vi "Graphics-Draw Line On Plot.vi"(8 "error in (no error)":errorcluster, 10 "X value":dbl, 11 "XYGraph in":refnum<vi>) -> (0 "error out":errorcluster)   [LabVIEW 2015]
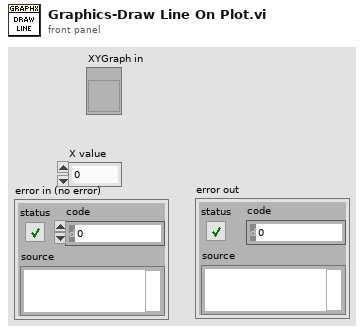
[diagram p1: front panel]
types:
  T1 = cluster{"Width":u16, "Style":enum32{"Solid", "Dash", "Dot", "DashDot", "DashDotDot"}}
  T2 = typedef "LVRectTypeDef.ctl" = cluster{"Left":i16, "Top":i16, "Right":i16, "Bottom":i16}
  T3 = typedef "LVPoint32TypeDef.ctl" = cluster{"Horizontal":i32, "Vertical":i32}
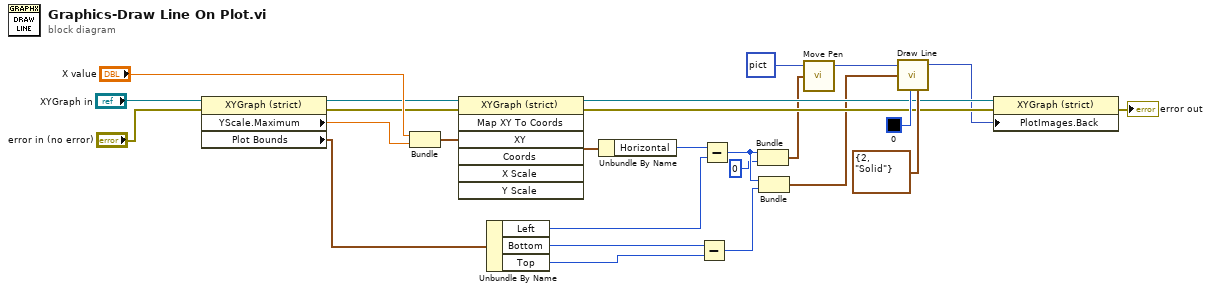
[diagram p0: block diagram]
diagram:
  n1 = property on="Property Node" class="XYGraph (strict)"(reference="XYGraph in", error in="error in (no error)") -> (reference out=w9:refnum<vi>, error out=w13:errorcluster, "YScale.Maximum"=w8:dbl, "Plot Bounds"=w21:T2)
  n2 = Bundle("X value"="X value", "YScale.Maximum"=w8) -> (w17:cluster{"X value":dbl, "YScale.Maximum":dbl})  [unwired: 1 in]
  n3 = invoke on="Invoke Node" class="XYGraph (strict)" method="Map XY To Coords"(reference=w9, error in=w13, "XY"=w17) -> (reference out=w14:refnum<vi>, error out=w15:errorcluster, "Coords"=w18:T3)  [unwired: 4 in, 4 out]
  n4 = Unbundle By Name(w21) -> ("Left"=w22:i16, "Bottom"=w1:i16, "Top"=w26:i16)
  n5 = Unbundle By Name(w18) -> ("Horizontal"=w7:i32)
  n6 = Subtract(x=w1, y=w26) -> (x-y=w5:i16)
  n7 = Subtract(x=w7, y=w22) -> (x-y=w6:i32)
  n8 = Bundle(w6, 0) -> (w4:cluster{i32, i32})  [unwired: 1 in]
  n9 = Bundle(w6, w5) -> (w3:cluster{i32, i16})  [unwired: 1 in]
  n10 = call <vilib>:"Move Pen.vi"("new position"=w4, "picture"=picture data[5B]) -> ("new picture"=w24:picture)  [unwired: 3 in]
  n11 = call <vilib>:"Draw Line.vi"("picture"=w24, "end point"=w3, "color(black)"=u32 0, "pen"=T1 {"Width"=2, "Style"=enum."Solid"}) -> ("new picture"=w12:picture)  [unwired: 5 in]
  n12 = property on="Property Node" class="XYGraph (strict)"(reference=w14, error in=w15, "PlotImages.Back"=w12) -> (error out=→"error out":errorcluster)  [unwired: 1 out]
